vi "NGTS_PID Parameters_VIG.vi"(7 "Operation":enum16{"get data", "set data", "initialize"}(ring)=enum."set data", 8 "error in":errorcluster, 11 "PID_Parameters In":T1[](array[typedef])=[{"Set Point (%)"=0.0, "PID_Gains"={"proportional gain (Kc)"=1.0, "integral time (Ti, min)"=0.01, "derivative time (Td, min)"=0.0}, "PID_Output_Range"={"OUTHI"=100.0, "OUTLO"=0.0}, "Mode"=FALSE, "Manual Value"=1.0, "PID_OK?"=FALSE, "Setpoint_Range"={"setpoint low"=0.0, "setpoint hi"=100.0}}] {"Setpoint_Range"."setpoint low" format="%.2f"; "Setpoint_Range"."setpoint hi" format="%.2f"; "Manual Value" format="%.3f"; "Set Point (%)" scale=0.0..100.0; "PID_Output_Range"."OUTLO" format="%.2f"; "PID_Output_Range"."OUTHI" format="%.2f"; "PID_Gains"."derivative time (Td, min)" format="%.3f"; "PID_Gains"."integral time (Ti, min)" format="%.3f"; "PID_Gains"."proportional gain (Kc)" format="%.3f"}) -> (0 "error out":errorcluster, 3 "PID_Parameters Out":T1[](array[typedef])=[{"Set Point (%)"=0.0, "PID_Gains"={"proportional gain (Kc)"=1.0, "integral time (Ti, min)"=0.01, "derivative time (Td, min)"=0.0}, "PID_Output_Range"={"OUTHI"=100.0, "OUTLO"=0.0}, "Mode"=FALSE, "Manual Value"=1.0, "PID_OK?"=FALSE, "Setpoint_Range"={"setpoint low"=0.0, "setpoint hi"=100.0}}] {"Setpoint_Range"."setpoint low" format="%.2f"; "Setpoint_Range"."setpoint hi" format="%.2f"; "Manual Value" format="%.3f"; "Set Point (%)" scale=0.0..100.0; "PID_Output_Range"."OUTLO" format="%.2f"; "PID_Output_Range"."OUTHI" format="%.2f"; "PID_Gains"."derivative time (Td, min)" format="%.3f"; "PID_Gains"."integral time (Ti, min)" format="%.3f"; "PID_Gains"."proportional gain (Kc)" format="%.3f"}, 4 "PID Param (Blank)":T1={"Set Point (%)"=0.0, "PID_Gains"={"proportional gain (Kc)"=1.0, "integral time (Ti, min)"=0.01, "derivative time (Td, min)"=0.0}, "PID_Output_Range"={"OUTHI"=100.0, "OUTLO"=0.0}, "Mode"=FALSE, "Manual Value"=1.0, "PID_OK?"=FALSE, "Setpoint_Range"={"setpoint low"=0.0, "setpoint hi"=100.0}} {"Setpoint_Range"."setpoint low" format="%.2f"; "Setpoint_Range"."setpoint hi" format="%.2f"; "Manual Value" format="%.3f"; "Set Point (%)" scale=0.0..100.0; "PID_Output_Range"."OUTLO" format="%.2f"; "PID_Output_Range"."OUTHI" format="%.2f"; "PID_Gains"."derivative time (Td, min)" format="%.3f"; "PID_Gains"."integral time (Ti, min)" format="%.3f"; "PID_Gains"."proportional gain (Kc)" format="%.3f"})   [LabVIEW 2010]
uses:
  PID_Parameters_TT.ctl
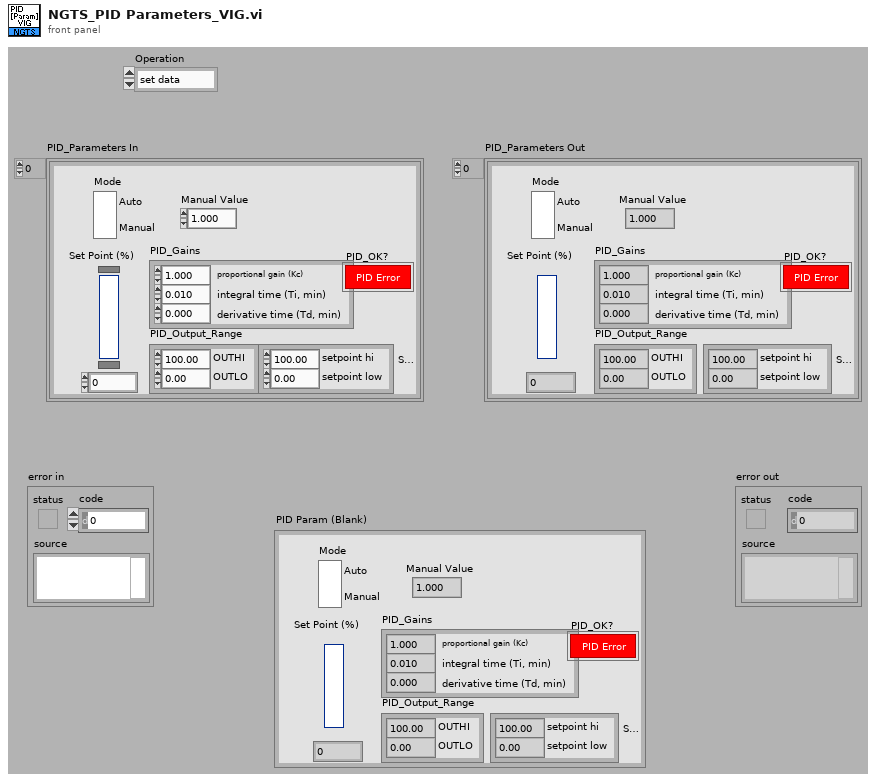
[diagram p1: front panel]
types:
  T1 = typedef "PID_Parameters_TT.ctl" = cluster{"Set Point (%)":dbl, "PID_Gains":cluster{"proportional gain (Kc)":dbl, "integral time (Ti, min)":dbl, "derivative time (Td, min)":dbl}, "PID_Output_Range":cluster{"OUTHI":dbl, "OUTLO":dbl}, "Mode":bool, "Manual Value":dbl, "PID_OK?":bool, "Setpoint_Range":cluster{"setpoint low":dbl, "setpoint hi":dbl}}
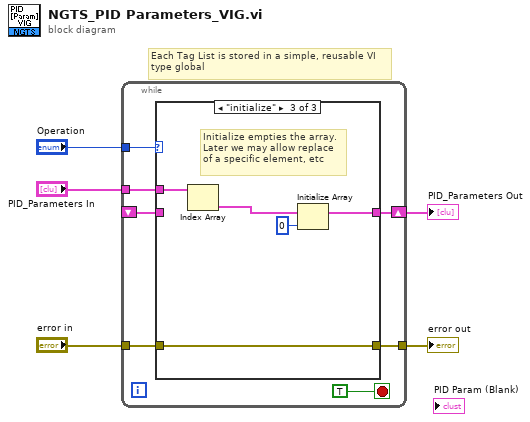
[diagram p0: block diagram]
diagram:
  # "Each Tag List is stored in a simple, reusable VI\ntype global"
  n1 = while {
    tunnel: "Operation" -> [w12]
    shift-right: [w10] -> w3
    shift-left: _ -> [w8]
    tunnel: "PID_Parameters In" -> [w9]
    tunnel: "error in" -> [w7]
    tunnel: [w6] -> w1
    stop <- TRUE stop-if-true
    n2 = case shown="\"initialize\"" w12 {
      tunnel: [w14 w16 w21] -> w10
      tunnel: w9 -> [_ w16 w19]
      tunnel: w8 -> [w14 _ _]
      tunnel: w7 -> [w13 w15 w20]
      tunnel: [w13 w15 w20] -> w6
      frame "get data", Default {
      }
      frame "set data" {
      }
      frame "initialize" {
        # "Initialize empties the array.\nLater we may allow replace\nof a specific element, etc"
        n3 = Index Array(array=w19) -> (element=w18:T1)  [unwired: 1 in]
        n4 = Initialize Array(w18, 0 ("dimension size")) -> (w21:T1[])
      }
    }
  }
  "error out" <- w1
  "PID_Parameters Out" <- w3
